vi "TCL Get Base Fragments - NeventNfrag.vi"(3 "error in (no error)":errorcluster, 4 "fragments":string[](array[string]), 5 "event numbers":i32[](array[numeric])) -> (0 "error out":errorcluster, 1 "values":string[][](array[string]), 2 "fragments out":string[](array[string]))   [LabVIEW 2010]
uses:
  TCL Global.vi
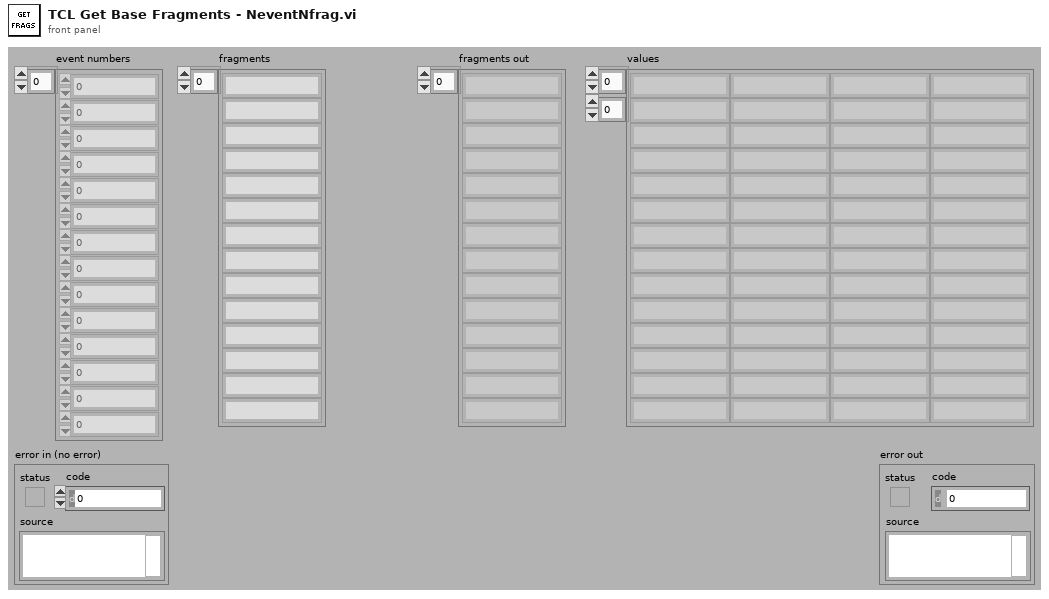
[diagram p1: front panel]
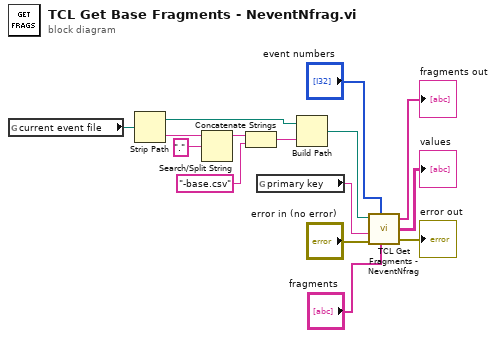
[diagram p0: block diagram]
diagram:
  n1 = global read "TCL Global.vi" "current event file"() -> (w9:path)
  n2 = Strip Path(path=w9) -> (stripped path=w3:path, name=w6:string)
  n3 = Search/Split String(string=w6, search string/char (-)=".") -> (substring before match=w4:string)  [unwired: 1 in, 2 out]
  n4 = Concatenate Strings(w4, "-base.csv" ("string")) -> (w2:string)
  n5 = global read "TCL Global.vi" "primary key"() -> (w8:string)
  n6 = Build Path(base path=w3, name or relative path=w2) -> (appended path=w1:path)
  n7 = call "TCL Get Fragments - NeventNfrag.vi"("event file"=w1, "event numbers"="event numbers", "primary key"=w8, "fragments"="fragments", "error in (no error)"="error in (no error)") -> ("fragments out"=→"fragments out":string[], "values"=→"values":string[][], "error out"=→"error out":errorcluster)  [unwired: 1 in]
